vi "222.vi"(0 "波形 I/Q 1":waveform(dbl)[](graph) caption="波形图 2") -> ()   [LabVIEW 2018]
uses:
  <vilib>/Waveform/WDTOps.llb/WDT Index Channel DBL.vi
  <vilib>/Utility/file.llb/Write Delimited Spreadsheet (DBL).vi
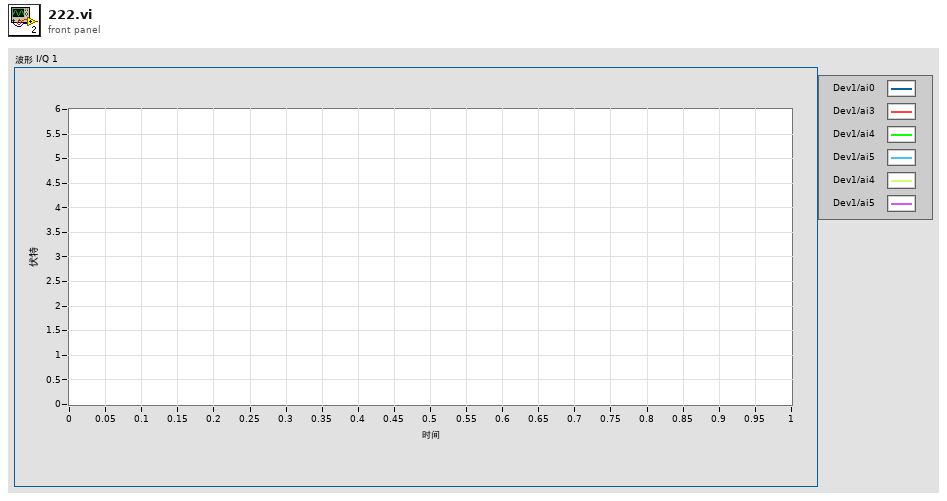
[diagram p1: front panel]
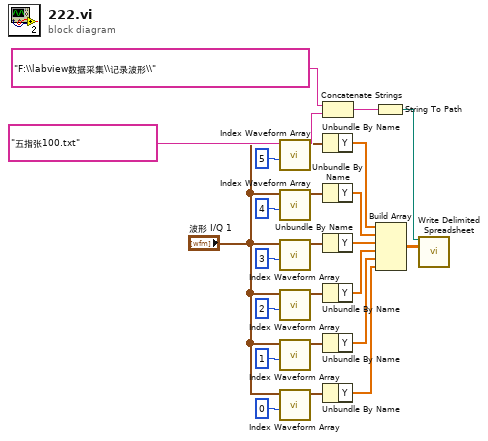
[diagram p0: block diagram]
diagram:
  n1 = call-poly <vilib>:"Index Waveform Array.vi"("index"=5, "waveform array"="波形 I/Q 1") -> ("waveform"=w19:waveform(dbl))  [unwired: 8 in, 1 out]
  n2 = call-poly <vilib>:"Index Waveform Array.vi"("index"=4, "waveform array"="波形 I/Q 1") -> ("waveform"=w18:waveform(dbl))  [unwired: 8 in, 1 out]
  n3 = call-poly <vilib>:"Index Waveform Array.vi"("index"=3, "waveform array"="波形 I/Q 1") -> ("waveform"=w9:waveform(dbl))  [unwired: 8 in, 1 out]
  n4 = call-poly <vilib>:"Index Waveform Array.vi"("index"=2, "waveform array"="波形 I/Q 1") -> ("waveform"=w8:waveform(dbl))  [unwired: 8 in, 1 out]
  n5 = call-poly <vilib>:"Index Waveform Array.vi"("index"=1, "waveform array"="波形 I/Q 1") -> ("waveform"=w7:waveform(dbl))  [unwired: 8 in, 1 out]
  n6 = call-poly <vilib>:"Index Waveform Array.vi"("index"=0, "waveform array"="波形 I/Q 1") -> ("waveform"=w6:waveform(dbl))  [unwired: 8 in, 1 out]
  n7 = Concatenate Strings("F:\\labview数据采集\\记录波形\\", "五指张100.txt" ("字符串")) -> (w1:string)
  n8 = Unbundle By Name(w19) -> ("Y"=w20:dbl[])
  n9 = Unbundle By Name(w18) -> ("Y"=w21:dbl[])
  n10 = Unbundle By Name(w9) -> ("Y"=w5:dbl[])
  n11 = Unbundle By Name(w8) -> ("Y"=w4:dbl[])
  n12 = Unbundle By Name(w7) -> ("Y"=w3:dbl[])
  n13 = Unbundle By Name(w6) -> ("Y"=w2:dbl[])
  n14 = String To Path(string=w1) -> (path=w22:path)
  n15 = Build Array(w20, w21, w5, w4, w3, w2) -> (w15:dbl[][])
  n16 = call-poly <vilib>:"Write Delimited Spreadsheet.vi"("file path (dialog if empty)"=w22, "2D data"=w15) -> ()  [unwired: 12 in, 2 out]
